vi "WPI_IMU_Loop.vi"(8 "error in":errorcluster, 11 "ADI IMU Interrupt DevRef":T1={"ADI IMU DevRef"={"DevStatus"={"status"=FALSE, "code"=0, "source"=""}, "Handle"=0, "SPI Bus"=enum."SPI On-Board, CS0", "Device Found"=FALSE, "Device Ready"=FALSE, "Yaw Axis"=enum."Z", "AHRS Algorithm"=enum."Complementary"}, "InterruptRef"={"DevStatus"={"status"=FALSE, "code"=0, "source"=""}, "InterruptIndex"=enum."0"}}) -> (0 "error out":errorcluster, 1 "Device Found":bool)   [LabVIEW 2015, in "FRC ADI MXP IMU.lvlib"]
doc: "Periodically reads the ADI MXP IMU valuse and makes data available for use elsewhere in your robot project. Place this block within PeriodicTasks.vi outside any loops."
uses:
  FRC ADI MXP IMU.lvlib
  WPI_AnalogDevicesIMUInterruptDevRef.ctl
  WPI_AnalogDevicesIMUDevRef.ctl
  <vilib>/Rock Robotics/SystemInterfaces/spilib/spi_bus.ctl
  <vilib>/Rock Robotics/WPI/Interrupt/WPI_InterruptRef.ctl
  <vilib>/Rock Robotics/SystemInterfaces/Interrupt/FPGA_InterruptIndex.ctl
  <vilib>/Rock Robotics/WPI/SPI/WPI_SPIDevRef.ctl
  <vilib>/Platform/TimedLoop/XDataNode/timing_clust.ctl
  <vilib>/Platform/TimedLoop/XDataNode/nitl_modes.ctl
  <vilib>/Platform/TimedLoop/XDataNode/wakeup.ctl
  <vilib>/Analysis/baseanly.llb/Mean (DBL).vi
  <vilib>/Rock Robotics/SystemInterfaces/Utilities/FPGA_UtilitiesRead LocalTime.vi
  <vilib>/Rock Robotics/SystemInterfaces/Interrupt/FPGA_WaitOnInterrupt.vi
  <vilib>/Rock Robotics/WPI/Utilities/WPI_UtilitiesTimebaseConstants.vi
  <vilib>/Rock Robotics/SystemInterfaces/Interrupt/FPGA_InterruptReadTimestamp.vi
  <vilib>/platform/TimedLoop/XDataNode/XDataNode.xnode
  <vilib>/Platform/TimedLoop/XDataNode/XDNodeRunTimeDep.lvlib
  <vilib>/Analysis/NI_AALBase.lvlib
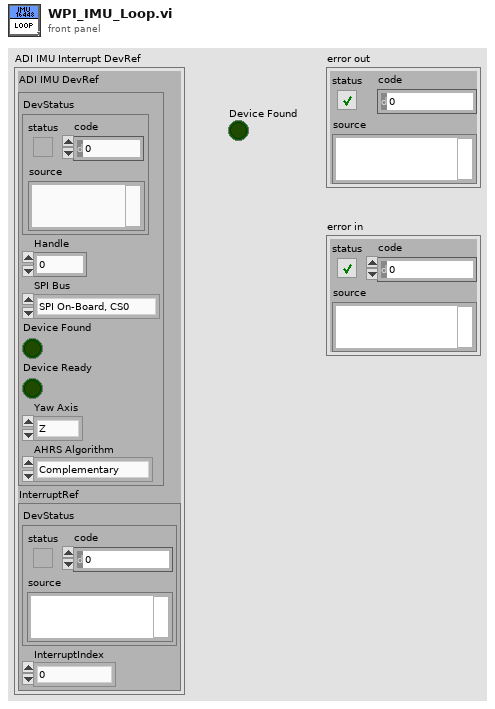
[diagram p1: front panel]
types:
  T1 = typedef "FRC ADI MXP IMU.lvlib/WPI_AnalogDevicesIMUInterruptDevRef.ctl" = cluster{"ADI IMU DevRef":T2, "InterruptRef":T4}
  T2 = typedef "FRC ADI MXP IMU.lvlib/WPI_AnalogDevicesIMUDevRef.ctl" = cluster{"DevStatus":errorcluster, "Handle":i32, "SPI Bus":T3, "Device Found":bool, "Device Ready":bool, "Yaw Axis":enum16{"X", "Y", "Z"}, "AHRS Algorithm":enum16{"Complementary", "Madgwick"}}
  T3 = typedef "spi_bus.ctl" = enum16{"SPI On-Board, CS0", "SPI On-Board, CS1", "SPI On-Board, CS2", "SPI On-Board, CS3", "SPI MXP", "Invalid"}
  T4 = typedef "WPI_InterruptRef.ctl" = cluster{"DevStatus":errorcluster, "InterruptIndex":T5}
  T5 = typedef "FPGA_InterruptIndex.ctl" = enum8{"0", "1", "2", "3", "4", "5", "6", "7", "Invalid"}
  T6 = typedef "WPI_SPIDevRef.ctl" = cluster{"DevStatus":errorcluster, "Handle":i32, "SPI Bus":T3}
  T7 = cluster{"X Angle":dbl, "Y Angle":dbl, "Z Angle":dbl}
  T8 = typedef "XDNodeRunTimeDep.lvlib/timing_clust.ctl" = cluster{"Expected End [f-1]":u64, "Actual End [f-1]":u64, "Finished Late? [f-1]":bool, "Expected End [i-1]":u64, "Actual End [i-1]":u64, "Finished Late? [i-1]":bool, "Expected Start [i]":u64, "Actual Start [i]":u64, "Expected Start [f]":u64, "Actual Start [f]":u64, "Source Name":string, "Structure Name":string, "Period":i64, "Deadline":i64, "Offset":i64, "Start":i64, "Priority":i32, "Timeout":i32, "Mode":T9, "Wakeup Reason":T10, "Error":errorcluster, "Source Type":string, "Secondary Source Type":string, "Global End Time":u64, "Global Start Time":u64, "Frame Duration":u64, "Iteration Duration":u64, "Assigned CPU":i32, "I/O Scan Engine Mode":u32}
  T9 = typedef "XDNodeRunTimeDep.lvlib/nitl_modes.ctl" = enum32{"No Change", "Process missed periods, maintain original phase", "Discard missed periods, maintain original phase", "Process missed periods, ignore original phase", "Discard missed periods, ignore original phase"}
  T10 = typedef "XDNodeRunTimeDep.lvlib/wakeup.ctl" = enum32{"Normal", "Aborted", "Asynchronous wakeup", "Timing source error", "Timed loop error", "Timeout"}
  T11 = cluster{"X Gyro":dbl, "Y Gyro":dbl, "Z Gyro":dbl, "X Accel":dbl, "Y Accel":dbl, "Z Accel":dbl, "X Mag":dbl, "Y Mag":dbl, "Z Mag":dbl, "Pressure":dbl, "Temp":dbl}
  T12 = cluster{"Output[0]":dbl, "Output[1]":dbl, "Output[2]":dbl}
  T13 = cluster{"appended array[0]":dbl, "appended array[1]":dbl, "appended array[2]":dbl}
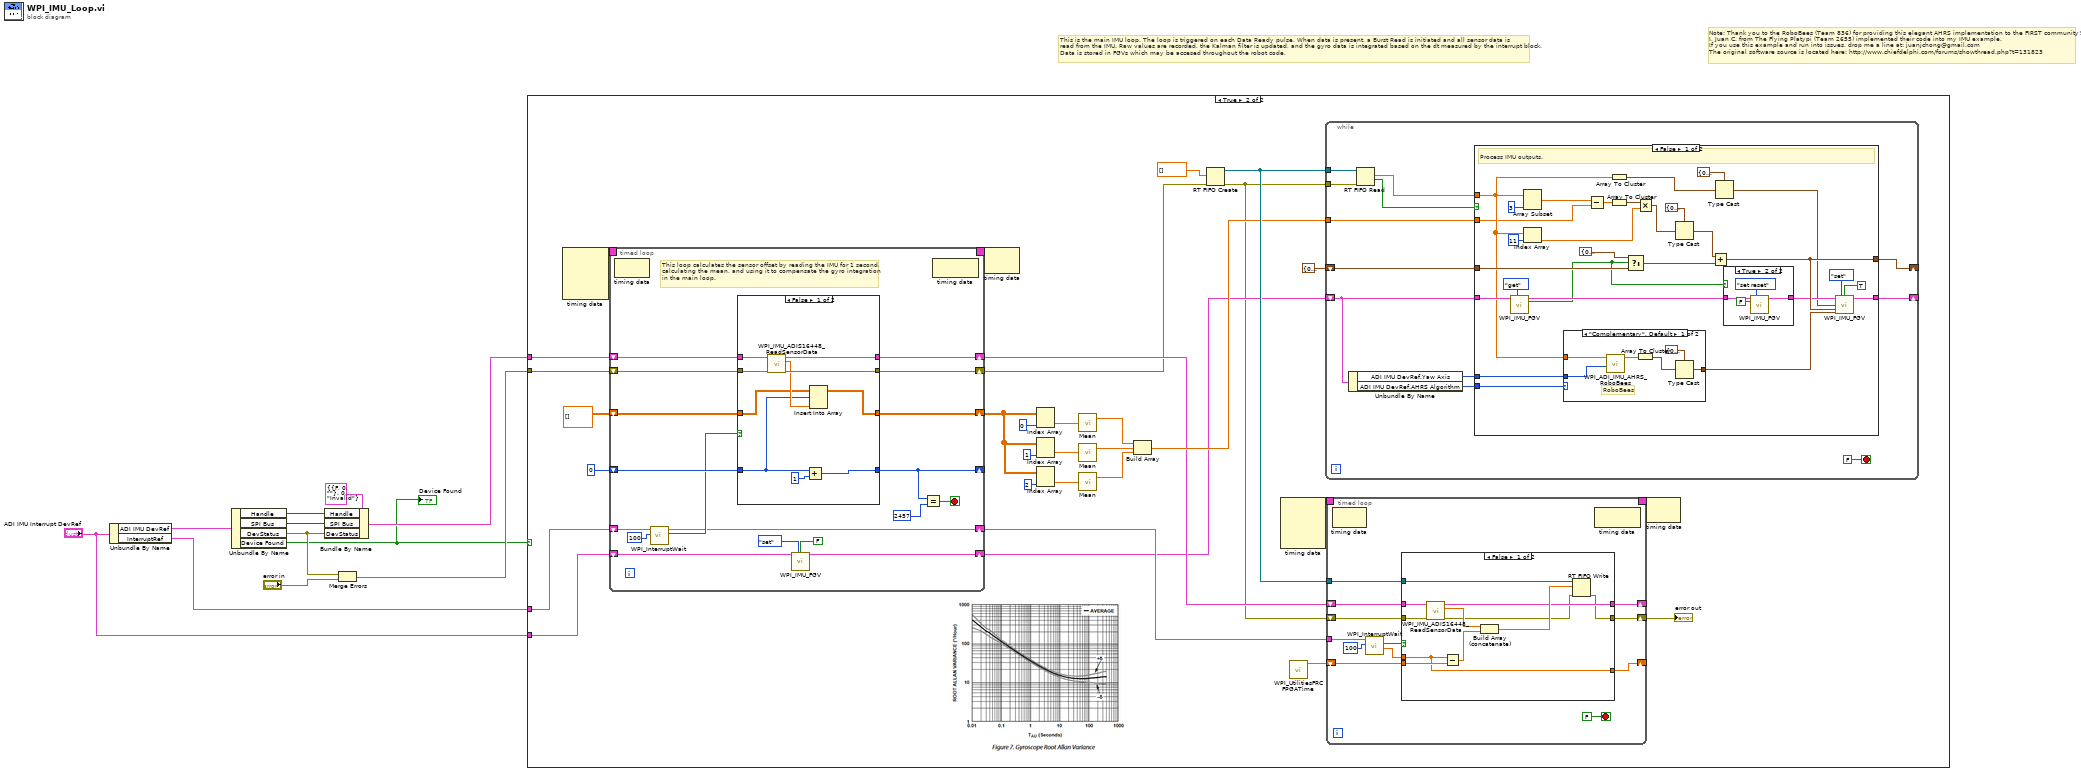
[diagram p0: block diagram]
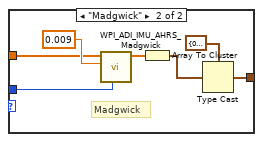
[diagram p4: hidden frame]
diagram:
  # "This is the main IMU loop. The loop is triggered on each Data Ready pulse. When data is present, a Burst Read is initiated and all sensor data is \nread from the IMU. Raw values are recorded, the Kalman filter is updated, and the gyro data is integrated based on the dt measured by the interrupt block.\nData is stored in FGVs which may be accesed throughout the robot code."
  # "Note: Thank you to the RoboBees (Team 836) for providing this elegant AHRS implementation to the FIRST community!\nI, Juan C. from The Flying Platypi (Team 2655) implemented their code into my IMU example.\nIf you use this example and run into issues, drop me a line at: juanjchong@gmail.com\nThe original software source is located here: http://www.chiefdelphi.com/forums/showthread.php?t=131823"
  n1 = Unbundle By Name("ADI IMU Interrupt DevRef") -> ("ADI IMU DevRef"=w7:T2, "InterruptRef"=w3:T4)
  n2 = Unbundle By Name(w7) -> ("Handle"=w10:i32, "SPI Bus"=w9:T3, "DevStatus"=w8:errorcluster, "Device Found"=w1:bool)
  "Device Found" <- w1
  n3 = Bundle By Name(cluster=T6 {"DevStatus"={"status"=FALSE, "code"=0, "source"=""}, "Handle"=0, "SPI Bus"=enum."Invalid"} ("SPIDevRef out"), "Handle"=w10, "SPI Bus"=w9, "DevStatus"=w8) -> (w5:T6)
  n4 = Merge Errors(w8, "error in") -> (w4:errorcluster)
  n5 = case shown="True" w1 {
    tunnel: w5 -> [_ w21]
    tunnel: w4 -> [_ w20]
    tunnel: w3 -> [_ w18]
    tunnel: "ADI IMU Interrupt DevRef" -> [_ w17]
    frame False {
    }
    frame True {
      n6 = node-c288() -> (w36:T8)  [unwired: 4 in]
      n7 = timed-loop {
        shift-right: [w59] -> w19
        shift-left: w21 -> [w54]
        shift-right: [w60] -> w14
        shift-left: w20 -> [w53]
        shift-right: [w49] -> _
        shift-left: 0 -> [w57]
        timing: w36 -> [_]
        timing-out: [_] -> w35
        shift-right: [w58] -> w30
        shift-left: dbl[][] [] -> [w51]
        shift-right: [w46] -> w16
        shift-left: w18 -> [w47]
        shift-right: [w45] -> w15
        shift-left: w17 -> [w44]
        stop <- w48 stop-if-true
        # "This loop calculates the sensor offset by reading the IMU for 1 second, \ncalculating the mean, and using it to compensate the gyro integration\nin the main loop."
        n8 = node-c288() -> ()  [unwired: 1 in, 1 out]
        n9 = call <vilib>:"WPI_InterruptWait.vi"("Timeout (ms)"=100, "InterruptRef"=w47) -> ("Timed Out"=w55:bool, "InterruptRef"=w46:T4)  [unwired: 5 in, 3 out]
        n10 = case shown="False" w55 {
          tunnel: [w72 w74] -> w60
          tunnel: [w71 w75] -> w59
          tunnel: [w63 w73] -> w58
          tunnel: w53 -> [w70 w74]
          tunnel: w54 -> [w69 w75]
          tunnel: w57 -> [w64 w76]
          tunnel: [w68 w76] -> w49
          tunnel: w51 -> [w65 w73]
          frame False {
            n11 = call "WPI_IMU_ADIS16448_ReadSensorData.vi"("error in (no error)"=w70, "SPIDevRef in"=w69) -> ("error out"=w72:errorcluster, "Data Array"=w66:dbl[], "SPIDevRef out"=w71:T6)  [unwired: 7 in]
            n12 = Add(x=w64, y=1) -> (x+y=w68:i32)
            n13 = Insert Into Array(array=w65, index (row)=w64, new element=w66) -> (w63:dbl[][])  [unwired: 1 in]
          }
          frame True {
          }
        }
        n14 = call "WPI_IMU_FGV.vi"("ADI IMU Interrupt DevRef"=w44, "Operation"=enum16{"set", "get", "set reset"}."set", "Sensor Ready?"=FALSE) -> ("ADI IMU Interrupt DevRef Out"=w45:T1)  [unwired: 6 in, 6 out]
        n15 = Equal?(x=w49, y=2457) -> (x = y?=w48:bool)
        n16 = node-c288() -> ()  [unwired: 1 in, 1 out]
      }
      n17 = node-c288(w35) -> ()  [unwired: 1 out]
      n18 = Index Array(array=w30, index (col)=0 ("disabled index (col)")) -> (element=w29:dbl[])  [unwired: 1 in]
      n19 = Index Array(array=w30, index (col)=1 ("disabled index (col)")) -> (element=w28:dbl[])  [unwired: 1 in]
      n20 = Index Array(array=w30, index (col)=2 ("disabled index (col)")) -> (element=w27:dbl[])  [unwired: 1 in]
      n21 = call-poly <vilib>:"Mean.vi"("X"=w29) -> ("mean"=w26:dbl)  [unwired: 1 out]
      n22 = call-poly <vilib>:"Mean.vi"("X"=w28) -> ("mean"=w25:dbl)  [unwired: 1 out]
      n23 = call-poly <vilib>:"Mean.vi"("X"=w27) -> ("mean"=w24:dbl)  [unwired: 1 out]
      n24 = Build Array(w26, w25, w24) -> (w22:dbl[])
      n25 = RT FIFO Create(1:dbl[] [] ("appended array"), 3:w14) -> (8:w39:refnum<k33>, 11:w13:errorcluster)  [unwired: 6 in, 1 out]
      n26 = node-c288() -> (w42:T8)  [unwired: 4 in]
      n27 = call <vilib>:"WPI_UtilitiesFRC FPGATime.vi"() -> ("FPGA Time"=w40:dbl)  [unwired: 10 in, 1 out]
      n28 = while {
        tunnel: w39 -> [w89]
        shift-right: [w84] -> _
        shift-left: T7 {"X Angle"=0.0, "Y Angle"=0.0, "Z Angle"=0.0} ("IMU Angles") -> [w85]
        shift-right: [w81] -> _
        shift-left: w15 -> [w80]
        tunnel: w22 -> [w79]
        tunnel: w13 -> [w88]
        stop <- FALSE stop-if-true
        n29 = Unbundle By Name(w80) -> ("ADI IMU DevRef.Yaw Axis"=w83:enum16{"X", "Y", "Z"}, "ADI IMU DevRef.AHRS Algorithm"=w82:enum16{"Complementary", "Madgwick"})
        n30 = RT FIFO Read(0:w89, 3:w88) -> (9:w86:dbl[], 10:w87:bool)  [unwired: 2 in, 3 out]
        n31 = case shown="False" w87 {
          tunnel: w86 -> [w96 _]
          tunnel: w85 -> [w112 w139]
          tunnel: [w110 w139] -> w84
          tunnel: w83 -> [w101 _]
          tunnel: w82 -> [w100 _]
          tunnel: w80 -> [w98 w138]
          tunnel: [w97 w138] -> w81
          tunnel: w79 -> [w92 _]
          frame False {
            # "Process IMU outputs."
            n32 = call "WPI_IMU_FGV.vi"("ADI IMU Interrupt DevRef"=w98, "Operation"=enum16{"set", "get", "set reset"}."get") -> ("ADI IMU Interrupt DevRef Out"=w104:T1, "Reset Out"=w103:bool)  [unwired: 7 in, 5 out]
            n33 = Array Subset(array=w96, length=3) -> (w118:dbl[])  [unwired: 1 in]
            n34 = Index Array(array=w96, index=11) -> (element=w102:dbl)
            n35 = case shown="\"Complementary\", Default" w100 {
              tunnel: w96 -> [w124 w130]
              tunnel: w101 -> [w123 w129]
              tunnel: [w120 w126] -> w99
              frame "Complementary", Default {
                # "RoboBees"
                n36 = call "WPI_ADI_IMU_AHRS_RoboBees.vi"("Yaw Axis"=w123, "IMU Rates"=w124) -> ("Output"=w125:dbl[])  [unwired: 5 in, 3 out]
                n37 = Array To Cluster(array=w125) -> (cluster=w121:T12)
                n38 = Type Cast(type=cluster{"Pitch":dbl, "Roll":dbl, "Yaw":dbl} {"Pitch"=0.0, "Roll"=0.0, "Yaw"=0.0} ("IMU AHRS"), x=w121) -> (*(type *) &x=w120:cluster{"Pitch":dbl, "Roll":dbl, "Yaw":dbl})
              }
              frame "Madgwick" {
                # "Madgwick"
                n39 = call "WPI_ADI_IMU_AHRS_Madgwick.vi"("Yaw Axis"=w129, "Beta"=0.009, "Data"=w130) -> ("Output"=w131:dbl[])  [unwired: 8 in]
                n40 = Array To Cluster(array=w131) -> (cluster=w127:T12)
                n41 = Type Cast(type=cluster{"Pitch":dbl, "Roll":dbl, "Yaw":dbl} {"Pitch"=0.0, "Roll"=0.0, "Yaw"=0.0} ("IMU AHRS"), x=w127) -> (*(type *) &x=w126:cluster{"Pitch":dbl, "Roll":dbl, "Yaw":dbl})
              }
            }
            n42 = Subtract(x=w118, y=w92) -> (x-y=w117:dbl[])
            n43 = Array To Cluster(array=w96) -> (cluster=w95:T13)
            n44 = Array To Cluster(array=w117) -> (cluster=w116:cluster{"[0]":dbl, "[1]":dbl, "[2]":dbl})
            n45 = Select(t=T7 {"X Angle"=0.0, "Y Angle"=0.0, "Z Angle"=0.0} ("IMU Angles"), s=w103, f=w112) -> (s? t:f=w114:T7)
            n46 = Multiply(x=w116, y=w102) -> (x*y=w107:cluster{"[0]":dbl, "[1]":dbl, "[2]":dbl})
            n47 = Type Cast(type=T7 {"X Angle"=0.0, "Y Angle"=0.0, "Z Angle"=0.0} ("IMU Angles"), x=w107) -> (*(type *) &x=w108:T7)
            n48 = Add(x=w108, y=w114) -> (x+y=w110:T7)
            n49 = Type Cast(type=T11 {"X Gyro"=0.0, "Y Gyro"=0.0, "Z Gyro"=0.0, "X Accel"=0.0, "Y Accel"=0.0, "Z Accel"=0.0, "X Mag"=0.0, "Y Mag"=0.0, "Z Mag"=0.0, "Pressure"=0.0, "Temp"=0.0} ("IMU Data"), x=w95) -> (*(type *) &x=w93:T11)
            n50 = case shown="True" w103 {
              tunnel: [w133 w136] -> w105
              tunnel: w104 -> [w133 w135]
              frame False {
              }
              frame True {
                n51 = call "WPI_IMU_FGV.vi"("ADI IMU Interrupt DevRef"=w135, "Operation"=enum16{"set", "get", "set reset"}."set reset", "Reset"=FALSE) -> ("ADI IMU Interrupt DevRef Out"=w136:T1)  [unwired: 6 in, 6 out]
              }
            }
            n52 = call "WPI_IMU_FGV.vi"("ADI IMU Interrupt DevRef"=w105, "Operation"=enum16{"set", "get", "set reset"}."set", "Sensor Ready?"=TRUE, "IMU Data"=w93, "IMU Angles"=w110, "IMU AHRS"=w99) -> ("ADI IMU Interrupt DevRef Out"=w97:T1)  [unwired: 3 in, 6 out]
          }
          frame True {
            # "No new data."
          }
        }
      }
      n53 = timed-loop {
        timing: w42 -> [_]
        timing-out: [_] -> w41
        shift-right: [w147] -> _
        shift-left: w40 -> [w148]
        tunnel: w39 -> [w146]
        shift-right: [w142] -> _
        shift-left: w19 -> [w144]
        shift-right: [w141] -> w12
        shift-left: w13 -> [w143]
        tunnel: w16 -> [w140]
        stop <- FALSE stop-if-true
        n54 = node-c288() -> ()  [unwired: 1 in, 1 out]
        n55 = call <vilib>:"WPI_InterruptWait.vi"("Timeout (ms)"=100, "InterruptRef"=w140) -> ("TimeStamp"=w149:dbl, "Timed Out"=w150:bool)  [unwired: 5 in, 3 out]
        n56 = case shown="False" w150 {
          tunnel: w149 -> [w160 _]
          tunnel: w148 -> [w161 w165]
          tunnel: [w160 w165] -> w147
          tunnel: w146 -> [w157 _]
          tunnel: w144 -> [w156 w164]
          tunnel: w143 -> [w155 w163]
          tunnel: [w154 w164] -> w142
          tunnel: [w152 w163] -> w141
          frame False {
            n57 = call "WPI_IMU_ADIS16448_ReadSensorData.vi"("error in (no error)"=w155, "SPIDevRef in"=w156) -> ("error out"=w153:errorcluster, "Data Array"=w162:dbl[], "SPIDevRef out"=w154:T6)  [unwired: 7 in]
            n58 = Subtract(x=w160, y=w161) -> (x-y=w159:dbl)
            n59 = Build Array (concatenate)(w162, w159) -> (w158:dbl[])
            n60 = RT FIFO Write(0:w157, 1:w158, 3:w153) -> (11:w152:errorcluster)  [unwired: 2 in, 3 out]
          }
          frame True {
          }
        }
        n61 = node-c288() -> ()  [unwired: 1 in, 1 out]
      }
      "error out" <- w12
      n62 = node-c288(w41) -> ()  [unwired: 1 out]
    }
  }
